vi "delete_col.vi"(11 "TO CSV. in":string[][](array[string])) -> (2 "element":i32, 3 "TO CSV. out":string[][](array[string]))   [LabVIEW 2017]
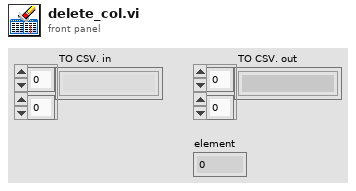
[diagram p1: front panel]
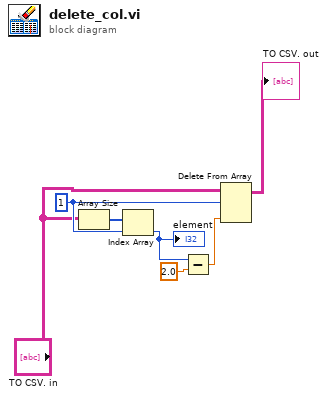
[diagram p0: block diagram]
diagram:
  w3 = 1 ("index")
  n1 = Array Size(array="TO CSV. in") -> (size(s)=w1:i32[])
  n2 = Index Array(array=w1, index=w3) -> (element=w6:i32)
  "element" <- w6
  n3 = Subtract(x=w6, y=2.0) -> (x-y=w7:dbl)
  n4 = Delete From Array(array="TO CSV. in", length=w3, index (col)=w7) -> (array with subset deleted=→"TO CSV. out":string[][])  [unwired: 1 in, 1 out]
